vi "LVPortFilterObjectMapNamepathDataByNamepathAndObjectType.vi"(6 "Object types":string[](array[string]), 9 "Namepaths":string[](array[string]), 10 "Variant":variant, 11 "Value Type (Or value to update)":variant) -> (3 "ObjectMap":T1[](array[typedef]))   [LabVIEW 2017]
uses:
  LVPortObjectMapNamepathData.ctl
  LVPortObjectMapDataTypeEnum.ctl
  LVPortObjectMapContainerTypeEnum.ctl
panel:
  in  "Object Map to compare to":T1[](array[typedef])
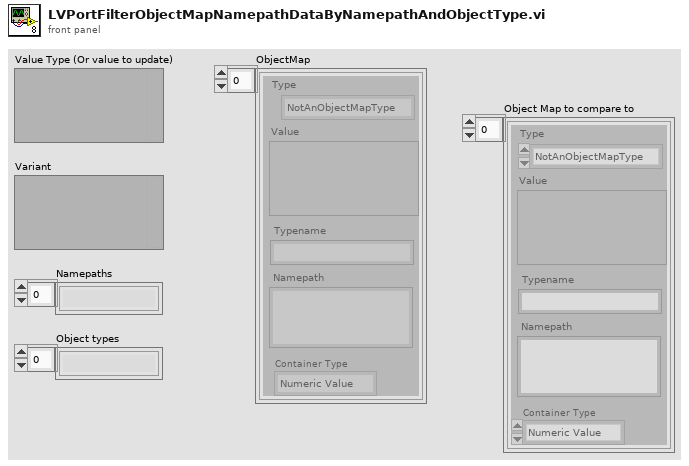
[diagram p1: front panel]
types:
  T1 = typedef "LVPortObjectMapNamepathData.ctl" = cluster{"Type":T2, "Value":variant, "Namepath":string, "Typename":string, "Container Type":T3}
  T2 = typedef "LVPortObjectMapDataTypeEnum.ctl" = enum16{"NotAnObjectMapType", "Real", "Complex", "String", "Boolean"}
  T3 = typedef "LVPortObjectMapContainerTypeEnum.ctl" = enum16{"Numeric Value", "Numeric Array", "Waveform"}
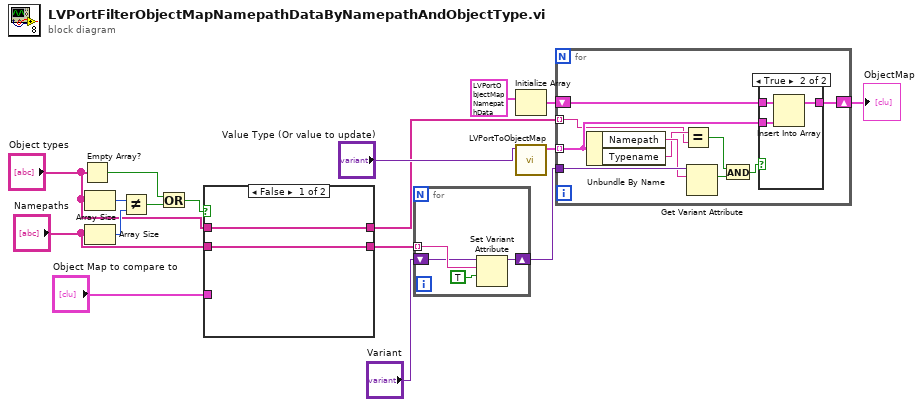
[diagram p0: block diagram]
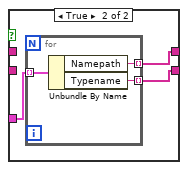
[diagram p2: hidden frame]
diagram:
  n1 = Empty Array?(array="Object types") -> (empty?=w7:bool)
  n2 = Array Size(array="Object types") -> (size(s)=w8:i32)
  n3 = Array Size(array="Namepaths") -> (size(s)=w9:i32)
  n4 = Not Equal?(x=w8, y=w9) -> (x != y?=w10:bool)
  n5 = Or(x=w7, y=w10) -> (x .or. y?=w6:bool)
  n6 = case shown="False" w6 {
    tunnel: "Object Map to compare to" -> [_ w22]
    tunnel: [w19 w21] -> w4
    tunnel: [w18 w20] -> w3
    tunnel: "Object types" -> [w19 _]
    tunnel: "Namepaths" -> [w18 _]
    frame False {
    }
    frame True {
      n7 = for {
        tunnel: w22 -> [w25] mode=indexing
        tunnel: [w24] -> w21 mode=indexing
        tunnel: [w23] -> w20 mode=indexing
        n8 = Unbundle By Name(w25) -> ("Namepath"=w24:string, "Typename"=w23:string)
      }
    }
  }
  n9 = for {
    tunnel: w3 -> [w29] mode=indexing
    shift-right: [w27] -> w15
    shift-left: "Variant" -> [w28]
    n10 = Set Variant Attribute(Variant=w28, name=w29, value=TRUE) -> (Variant out=w27:variant)  [unwired: 1 in, 2 out]
  }
  n11 = Initialize Array(T1 {"Type"=enum."NotAnObjectMapType", "Value"=variant, "Namepath"="", "Typename"="", "Container Type"=enum."Numeric Value"} ("ObjectMap")) -> (w14:T1[])  [unwired: 1 in]
  n12 = call "LVPortToObjectMap.vi"("Value"="Value Type (Or value to update)") -> ("Object map"=w16:T1[])  [unwired: 10 in]
  n13 = for {
    shift-right: [w36] -> w17
    shift-left: w14 -> [w37]
    tunnel: w15 -> [w39]
    tunnel: w16 -> [w35] mode=indexing
    tunnel: w4 -> [w33] mode=indexing
    n14 = Unbundle By Name(w35) -> ("Namepath"=w38:string, "Typename"=w34:string)
    n15 = Equal?(x=w34, y=w33) -> (x = y?=w32:bool)
    n16 = Get Variant Attribute(Variant=w39, name=w38) -> (found=w31:bool)  [unwired: 2 in, 3 out]
    n17 = And(x=w32, y=w31) -> (x .and. y?=w30:bool)
    n18 = case shown="True" w30 {
      tunnel: w37 -> [w40 w43]
      tunnel: [w40 w42] -> w36
      tunnel: w35 -> [_ w41]
      frame False {
      }
      frame True {
        n19 = Insert Into Array(array=w43, new element=w41) -> (w42:T1[])  [unwired: 1 in]
      }
    }
  }
  "ObjectMap" <- w17
